vi "stateMachine.vi"() -> ()   [LabVIEW 2020]
uses:
  C:/Users/DESKTOP-TLO0G68A/Desktop/LabVIEW/instrumentationLV/Thorlabs.MotionControl.Controls.dll
  Thorlabs.MotionControl.Controls.dll
  C:/Users/DESKTOP-TLO0G68A/Desktop/LabVIEW/instrumentationLV/ThorLabs.MotionControl.KCube.DCServoCLI.dll
  ThorLabs.MotionControl.KCube.DCServoCLI.dll
  C:/Users/DESKTOP-TLO0G68A/Desktop/LabVIEW/instrumentationLV/Thorlabs.MotionControl.GenericMotorCLI.dll
  Thorlabs.MotionControl.GenericMotorCLI.dll
panel:
  out "current y":i32
  out "current x":i32
  in  "y steps":i32
  in  "stepSize":dbl
  in  "x steps":i32
  in  "SerialNumber 2":string="27250520"
  in  "KCubeDCServoControl 2":refnum<k24>(container)
  in  "Begin Scan":bool
  in  "SerialNumber":string="27502753"
  in  "KCubeDCServoControl":refnum<k24>(container)
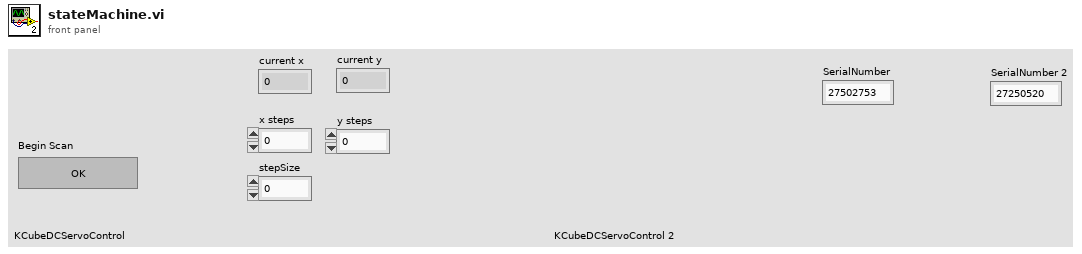
[diagram p1: front panel]
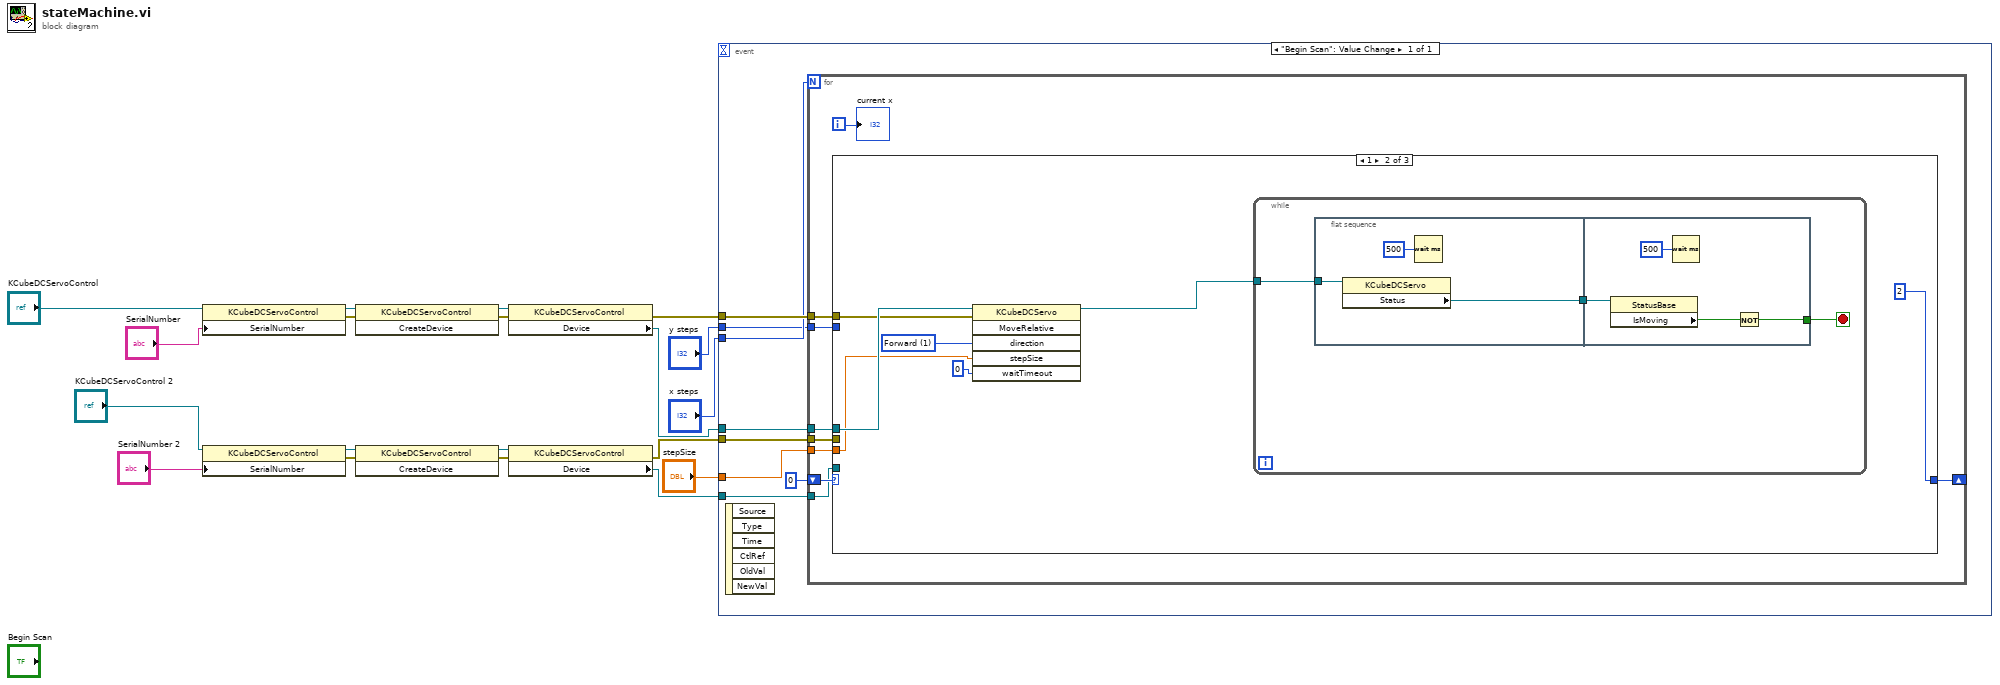
[diagram p0: block diagram]
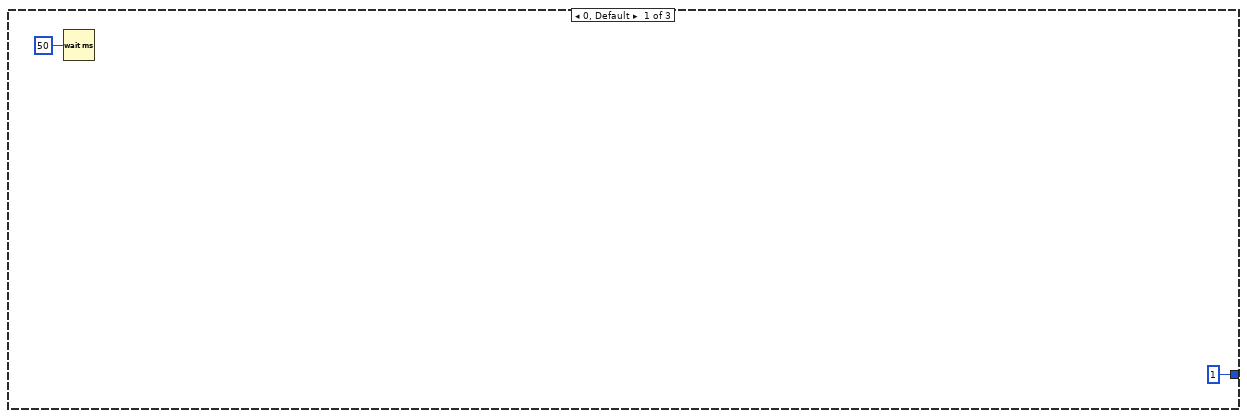
[diagram p2: hidden frame]
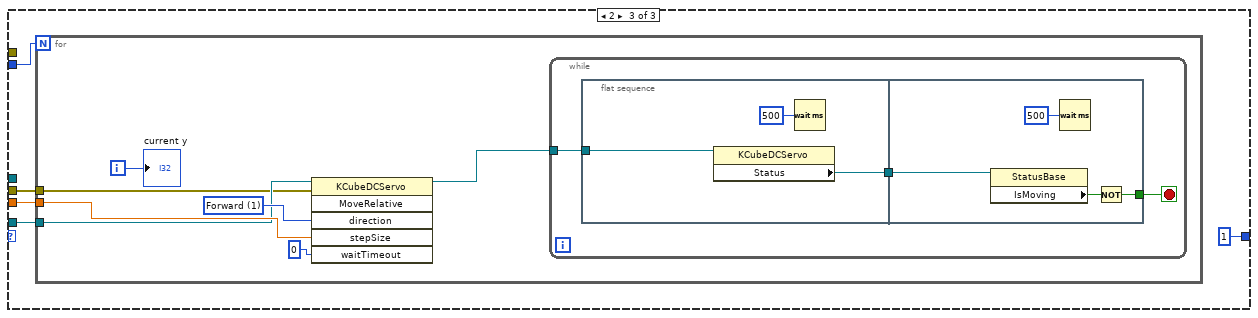
[diagram p3: hidden frame]
diagram:
  n1 = property class="KCubeDCServoControl"(reference="KCubeDCServoControl", "SerialNumber"="SerialNumber") -> (reference out=w18:refnum<k24>, error out=w16:errorcluster)  [unwired: 1 in]
  n2 = property class="KCubeDCServoControl"(reference="KCubeDCServoControl 2", "SerialNumber"="SerialNumber 2") -> (reference out=w12:refnum<k24>, error out=w10:errorcluster)  [unwired: 1 in]
  n3 = invoke class="KCubeDCServoControl" method="CreateDevice"(reference=w18, error in=w16) -> (reference out=w17:refnum<k24>, error out=w15:errorcluster)  [unwired: 1 in, 1 out]
  n4 = invoke class="KCubeDCServoControl" method="CreateDevice"(reference=w12, error in=w10) -> (reference out=w11:refnum<k24>, error out=w9:errorcluster)  [unwired: 1 in, 1 out]
  n5 = property class="KCubeDCServoControl"(reference=w17, error in=w15) -> (error out=w7:errorcluster, "Device"=w6:refnum<k24>)  [unwired: 1 out]
  n6 = property class="KCubeDCServoControl"(reference=w11, error in=w9) -> (error out=w4:errorcluster, "Device"=w5:refnum<k24>)  [unwired: 1 out]
  n7 = event shown="[0] \"Begin Scan\": Value Change" {
    selector: _ -> [_]
    dyn-events: _ -> [_]
    timeout: _ -> [_]
    tunnel: w7 -> [w27]
    tunnel: w6 -> [w26]
    tunnel: w5 -> [w25]
    tunnel: w4 -> [w24]
    tunnel: "x steps" -> [w22]
    tunnel: "y steps" -> [w21]
    tunnel: "stepSize" -> [w20]
    event "Begin Scan": Value Change {
      n8 = event-data() -> ()  [unwired: 1 in, 6 out]
      n9 = for {
        N: w22 -> [_]
        shift-right: [w29] -> _
        shift-left: 0 -> [w36]
        tunnel: w20 -> [w35]
        tunnel: w26 -> [w34]
        tunnel: w27 -> [w33]
        tunnel: w21 -> [w32]
        tunnel: w25 -> [w31]
        tunnel: w24 -> [w30]
        i -> [w28]
        n10 = case shown="1" w36 {
          tunnel: w35 -> [_ w44 w60]
          tunnel: w34 -> [_ w45 _]
          tunnel: w33 -> [_ w40 _]
          tunnel: w32 -> [_ _ w57]
          tunnel: w31 -> [_ _ w59]
          tunnel: w30 -> [_ _ w58]
          tunnel: [1 2 1] -> w29
          frame 0, Default {
            n11 = Wait (ms)(milliseconds to wait=u32 50) -> ()  [unwired: 1 out]
          }
          frame 1 {
            w43 = 1 items=["Forward"=1, "Backward"=2] ("direction")
            n12 = invoke class="KCubeDCServo" method="MoveRelative"(reference=w45, error in=w40, "direction"=w43, "stepSize"=w44, "waitTimeout"=0) -> (reference out=w41:refnum<k24>)  [unwired: 1 in, 5 out]
            n13 = while {
              tunnel: w41 -> [w47]
              stop <- w46 stop-if-true
              n14 = flat-sequence {
                tunnel: w47 -> [w51]
                tunnel: [w49] -> w48
                tunnel: [w52] -> w46
                tunnel: w48 -> [w54]
                frame #0 {
                  n15 = property class="KCubeDCServo"(reference=w51) -> ("Status"=w49:refnum<k24>)  [unwired: 1 in, 2 out]
                  n16 = Wait (ms)(milliseconds to wait=500) -> ()  [unwired: 1 out]
                }
                frame #1 {
                  n17 = property class="StatusBase"(reference=w54) -> ("IsMoving"=w53:bool)  [unwired: 1 in, 2 out]
                  n18 = Wait (ms)(milliseconds to wait=500) -> ()  [unwired: 1 out]
                  n19 = Not(x=w53) -> (.not. x?=w52:bool)
                }
              }
            }
          }
          frame 2 {
            n20 = for {
              N: w57 -> [_]
              tunnel: w60 -> [w64]
              tunnel: w59 -> [w63]
              tunnel: w58 -> [w62]
              i -> [w61]
              w67 = 1 items=["Forward"=1, "Backward"=2] ("direction")
              n21 = invoke class="KCubeDCServo" method="MoveRelative"(reference=w63, error in=w62, "direction"=w67, "stepSize"=w64, "waitTimeout"=0) -> (reference out=w65:refnum<k24>)  [unwired: 1 in, 5 out]
              n22 = while {
                tunnel: w65 -> [w69]
                stop <- w68 stop-if-true
                n23 = flat-sequence {
                  tunnel: w69 -> [w73]
                  tunnel: [w71] -> w70
                  tunnel: w70 -> [w76]
                  tunnel: [w74] -> w68
                  frame #0 {
                    n24 = property class="KCubeDCServo"(reference=w73) -> ("Status"=w71:refnum<k24>)  [unwired: 1 in, 2 out]
                    n25 = Wait (ms)(milliseconds to wait=500) -> ()  [unwired: 1 out]
                  }
                  frame #1 {
                    n26 = property class="StatusBase"(reference=w76) -> ("IsMoving"=w75:bool)  [unwired: 1 in, 2 out]
                    n27 = Wait (ms)(milliseconds to wait=500) -> ()  [unwired: 1 out]
                    n28 = Not(x=w75) -> (.not. x?=w74:bool)
                  }
                }
              }
              "current y" <- w61
            }
          }
        }
        "current x" <- w28
      }
    }
  }
